vi "initialize.vi"(0 "NInstrSim_ConfigureWaveformType":refnum<class "NInstrSim_ConfigureWaveformType.lvclass">, 3 "initializationData":variant, 5 "error in (no error)":errorcluster, 7 "binaryString":string, 8 "I8 Array":i8[](array[numeric]), 9 "prependSize? (T)":bool, 11 "byteOrder (0:big-endian, network order)":T1(ring)) -> (14 "dup NInstrSim_ConfigureWaveformType":refnum<class "NInstrSim_ConfigureWaveformType.lvclass">, 17 "found?":bool, 19 "error out":errorcluster)   [LabVIEW 2009, in "HB_Device_Examples.lvlib" / "NInstrSim_ConfigureWaveformType.lvclass"]
doc: "This is a dynamic dispatch VI to be implemented by child classes to initialize their attributes.\n\n<B>Recommendation:</B> Use Variant for initialization data."
uses:
  NInstrSim_ConfigureWaveformType.lvclass
  NInstrSim_Visitor.lvclass
  NInstrSim_ConfigureWaveformType.lvclass/NInstrSim_ConfigureWaveformType.ctl
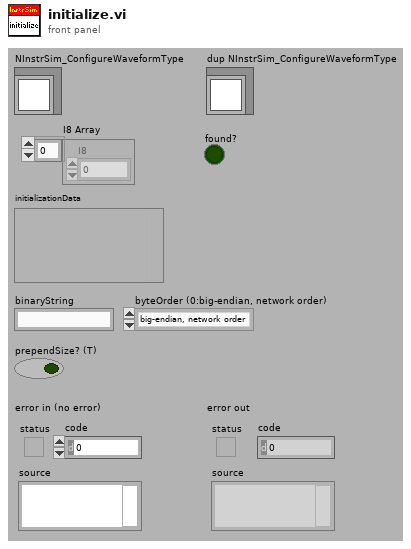
[diagram p1: front panel]
types:
  T1 = enum16{"big-endian, network order", "native, host order", "little-endian"}
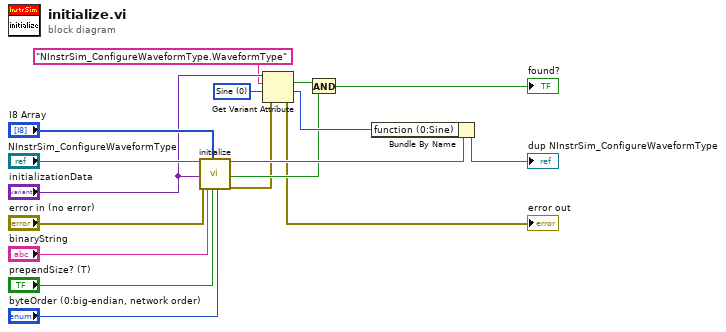
[diagram p0: block diagram]
diagram:
  w2 = u16 0 items=["Sine", "Square", "Sine+Noise", "Random", "Chirp"] ("function (0:Sine)")
  n1 = call-parent "initialize.vi"("HGF_NetworkData"="NInstrSim_ConfigureWaveformType", "initializationData"="initializationData", "error in (no error)"="error in (no error)", "binaryString"="binaryString", "I8 Array"="I8 Array", "prependSize? (T)"="prependSize? (T)", "byteOrder (0:big-endian, network order)"="byteOrder (0:big-endian, network order)") -> ("dup HGF_NetworkData"=w10:refnum<class "NInstrSim_ConfigureWaveformType.lvclass">, "found?"=w6:bool, "error out"=w4:errorcluster)  [unwired: 10 out]
  n2 = Get Variant Attribute(Variant="initializationData", name="NInstrSim_ConfigureWaveformType.WaveformType", default value (empty Variant)=w2, error in=w4) -> (found=w7:bool, value=w8:u16, error out=→"error out":errorcluster)  [unwired: 1 out]
  n3 = And(x=w7, y=w6) -> (x .and. y?=→"found?":bool)
  n4 = Bundle By Name(cluster=w10, "function (0:Sine)"=w8) -> (→"dup NInstrSim_ConfigureWaveformType":refnum<class "NInstrSim_ConfigureWaveformType.lvclass">)
